vi "GetMonitorResolution.vi"() -> ()   [LabVIEW 2017]
uses:
  user32.dll
panel:
  out "Array 2":i32[](array[numeric])
  out "error out":errorcluster
  in  "error in (no error)":errorcluster
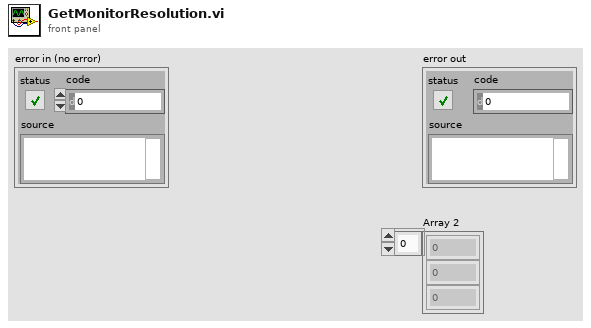
[diagram p1: front panel]
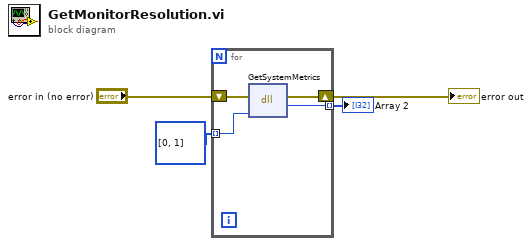
[diagram p0: block diagram]
diagram:
  n1 = for {
    tunnel: i32[] [0, 1] ("nIndex") -> [w7] mode=indexing
    tunnel: [w5] -> w1 mode=indexing
    shift-right: [w6] -> w2
    shift-left: "error in (no error)" -> [w8]
    n2 = dll-call lib="user32.dll" fn="GetSystemMetrics"(error in=w8, "nIndex"=w7) -> (error out=w6:errorcluster, "return type"=w5:i32)  [unwired: 3 in, 1 out]
  }
  "error out" <- w2
  "Array 2" <- w1
